vi "Write state.vi"(8 "error in (no error)":errorcluster, 10 "state":T1, 11 "MB in":refnum<class "Modbus Master CR.lvclass">) -> (0 "error out":errorcluster, 3 "MB out":refnum<class "Modbus Master CR.lvclass">)   [LabVIEW 2021, in "Modbus Master CR.lvclass"]
uses:
  Modbus Master CR.lvclass
  ctl/MB_TCP_State.ctl
  Modbus Master CR.lvclass/Modbus Master CR.ctl
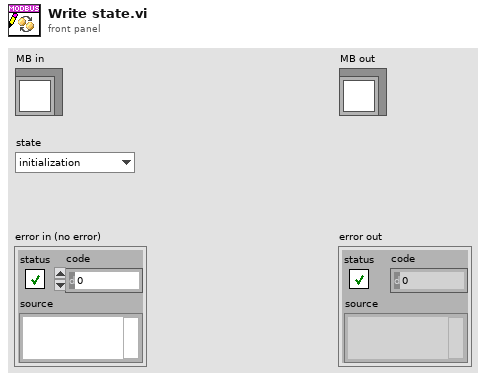
[diagram p1: front panel]
types:
  T1 = typedef "Modbus Master CR.lvclass/MB_TCP_State.ctl" = enum8{"initialization", "redefine", "standby", "ping", "connect", "wait to reconnect", "wait to reset timeout", "configure", "requests", "close connection", "stop"}
  T2 = typedef "Modbus Master CR.lvclass/MB state.ctl" = cluster{"state":T3, "enable":bool, "Run":bool, "write enable":bool, "Write":bool, "connect":bool, "errors":i32}
  T3 = typedef "MB_v2.lvlib/Modbus Master CR.lvclass/MB_TCP_State.ctl" = enum8{"initialization", "redefine", "standby", "ping", "connect", "wait to reconnect", "wait to reset timeout", "configure", "requests", "close connection", "stop"}
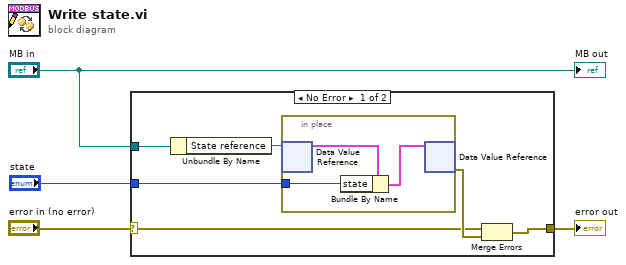
[diagram p0: block diagram]
diagram:
  n1 = case shown="No Error" "error in (no error)" {
    selector: "error in (no error)" -> [w5 w14]
    tunnel: [w7 w14] -> w3
    tunnel: "MB in" -> [w6 _]
    tunnel: "state" -> [w9 _]
    frame No Error {
      n2 = Unbundle By Name(w6) -> ("State reference"=w10:refnum<data-value>)
      n3 = in-place {
        in-place-border: w9 -> [w11]
        n4 = in-place-dvr #1(w10) -> (w13:T2)  [unwired: 1 out]
        n5 = Bundle By Name(cluster=w13, "state"=w11) -> (w12:T2)
        n6 = in-place-dvr #1(w12) -> (w8:errorcluster)  [unwired: 1 out]
      }
      n7 = Merge Errors(w5, w8) -> (w7:errorcluster)
    }
    frame Error {
    }
  }
  "error out" <- w3
  "MB out" <- "MB in"
